vi "SDT_AddCheckSum.vi"(11 "bhfile_header":T1 {"chksum" format="x%x"; "header_valid" format="x%x"}) -> (2 "Checksum":u16 format="%04x", 3 "HeaderWithChkSum":T1 {"chksum" format="x%x"; "header_valid" format="x%x"})   [LabVIEW 2017]
doc: "Use this VI to calculate and insert the correct U16 chksum into the bhfile_header cluster when writing a SDT- or SET-file.\nThe sum over all bhfile_header's words needs to add up to x55AA with overflow ignored.\n\ninfo@becker-hickl.com"
uses:
  SPC_Wrappers/SPC_Controls/bhfile_header.ctl
panel:
  out "u8 Array":u8[](array[numeric])
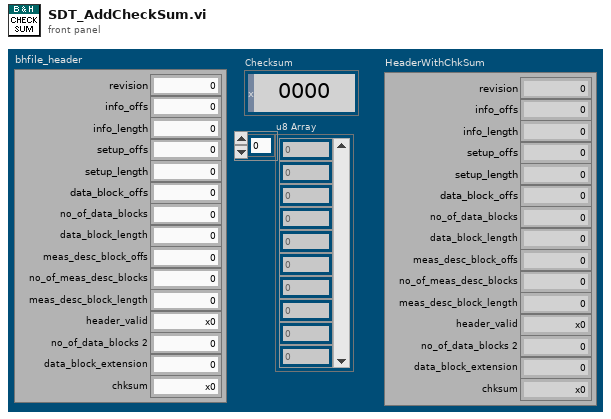
[diagram p1: front panel]
types:
  T1 = typedef "bhfile_header.ctl" = cluster{"revision":i16, "info_offs":i32, "info_length":i16, "setup_offs":i32, "setup_length":u16, "data_block_offs":i32, "no_of_data_blocks":i16, "data_block_length":u32, "meas_desc_block_offs":i32, "no_of_meas_desc_blocks":i16, "meas_desc_block_length":i16, "header_valid":u16, "no_of_data_blocks 2":u32, "data_block_extension":u16, "chksum":u16}
  T2 = enum16{"big-endian, network order", "native, host order", "little-endian"}
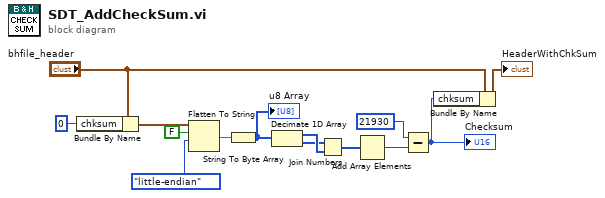
[diagram p0: block diagram]
diagram:
  n1 = Bundle By Name(cluster="bhfile_header", "chksum"=u16 0) -> (w4:T1)
  n2 = Flatten To String(anything=w4, prepend array or string size? (T)=FALSE, byte order (0:big-endian, network order)=T2."little-endian") -> (data string=w8:string)  [unwired: 1 in, 2 out]
  n3 = String To Byte Array(string=w8) -> (unsigned byte array=w3:u8[])
  "u8 Array" <- w3
  n4 = Decimate 1D Array(w3) -> (w12:u8[], w11:u8[])
  n5 = Join Numbers(hi=w11, lo=w12) -> ((hi.lo)=w10:u16[])
  n6 = Add Array Elements(numeric array=w10) -> (sum=w14:u16)
  n7 = Subtract(x=u16 21930, y=w14) -> (x-y=w1:u16)
  "Checksum" <- w1
  n8 = Bundle By Name(cluster="bhfile_header", "chksum"=w1) -> (→"HeaderWithChkSum":T1)
